vi "Read SV.vi"(8 "error in (no error)":errorcluster, 10 "Data":dbl[](array[numeric]), 11 "Read Refs by Type":cluster{"DBL Read":refnum<k21>[]}) -> (0 "error out":errorcluster, 2 "Data Out":dbl[](array[numeric]))   [LabVIEW 2020, in "Shared Variable Interface.lvlib"]
uses:
  Shared Variable Interface.lvlib
  DataTypes/DBL.lvlib
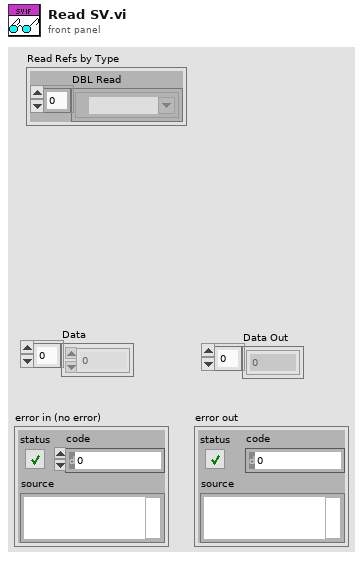
[diagram p1: front panel]
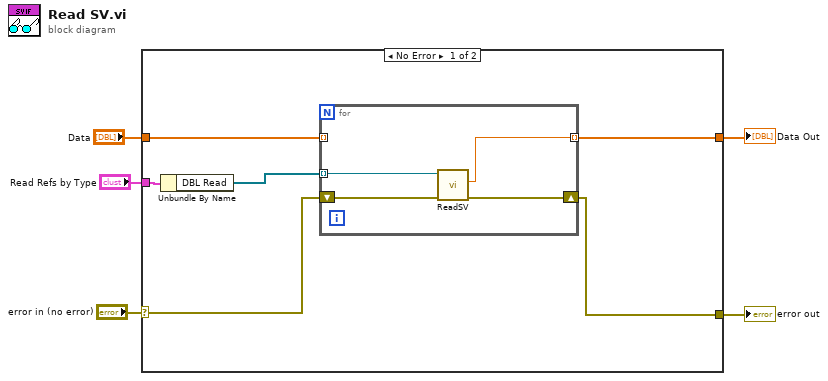
[diagram p0: block diagram]
diagram:
  n1 = case shown="No Error" "error in (no error)" {
    selector: "error in (no error)" -> [w9 w17]
    tunnel: [w8 w17] -> w5
    tunnel: "Data" -> [w7 w16]
    tunnel: [w6 w16] -> w3
    tunnel: "Read Refs by Type" -> [w10 _]
    frame No Error {
      n2 = Unbundle By Name(w10) -> ("DBL Read"=w11:refnum<k21>[])
      n3 = for {
        shift-right: [w14] -> w8
        shift-left: w9 -> [w15]
        tunnel: w11 -> [w13] mode=indexing
        tunnel: w7 -> [_] mode=indexing
        tunnel: [w12] -> w6 mode=indexing
        n4 = call "ReadSV.vi"("error in (no error)"=w15, "shared variable refnum"=w13) -> ("error out"=w14:errorcluster, "DBL Data"=w12:dbl)  [unwired: 8 in]
      }
    }
    frame Error {
    }
  }
  "error out" <- w5
  "Data Out" <- w3
